vi "MasterStateController.vi"(1 "Selected State (In)":string) -> (0 "Selected State (Out)":string)   [LabVIEW 2019]
uses:
  6eb6b6c3-9e30-4625-8a84-628f4f349f2d.vi
  6eb6b6c3-9e30-4625-8a84-628f4f349f2d.vi/f3f6f8f9-418a-4164-be9e-b0b809c44121.vi
  dsdata.vi
  constants.vi
  outputs.vi
  <vilib>/Rock Robotics/Network Tables/NT Write Value.vi
  <vilib>/Rock Robotics/Network Tables/NT Write String.vi
panel:
  out "State Index":i32
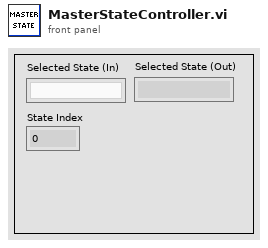
[diagram p1: front panel]
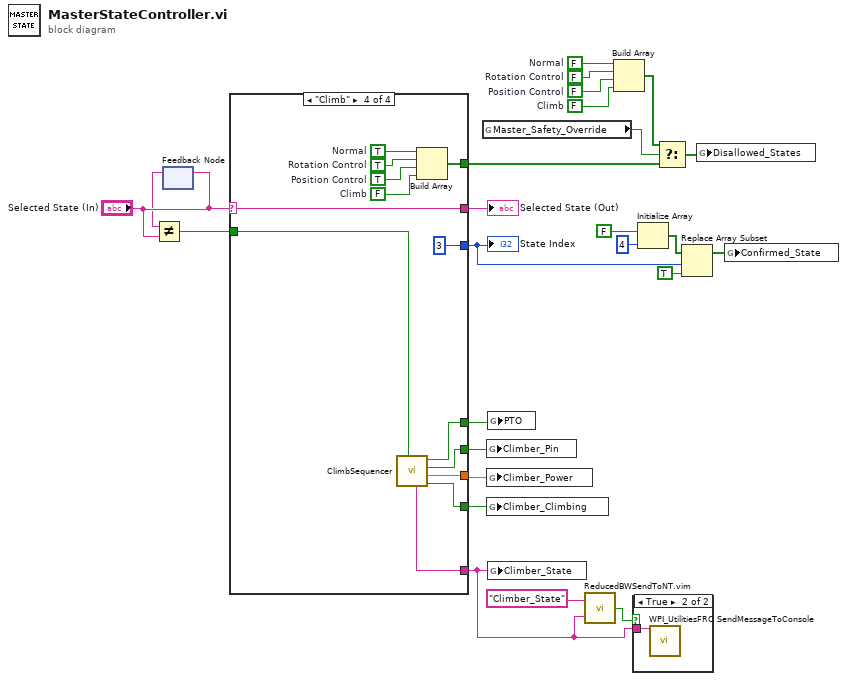
[diagram p0: block diagram]
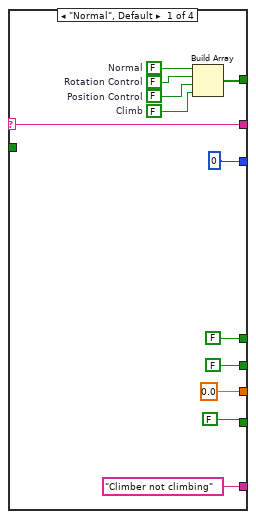
[diagram p3: hidden frame]
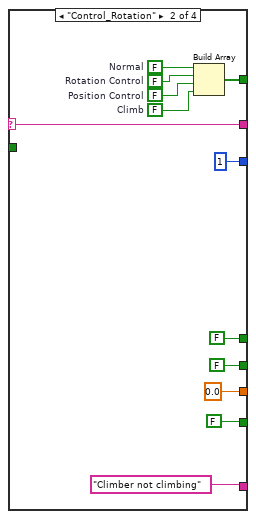
[diagram p4: hidden frame]
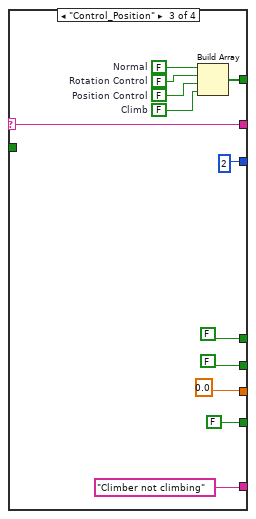
[diagram p5: hidden frame]
diagram:
  w12 = FALSE  # Climb
  w14 = FALSE  # Rotation Control
  w13 = FALSE  # Position Control
  w15 = FALSE  # Normal
  n1 = feedback-in #1("Selected State (In)") -> ()
  n2 = feedback #1() -> (w6:string)  [unwired: 1 in]
  n3 = Not Equal?(x=w6, y="Selected State (In)") -> (x != y?=w5:bool)
  n4 = case shown="\"Climb\"" "Selected State (In)" {
    selector: "Selected State (In)" -> [w36 w48 w61 w73]
    tunnel: [0 ("Index") 1 ("Index") 2 ("Index") 3 ("Index")] -> w22
    tunnel: [w36 w48 w61 w73] -> w19
    tunnel: [0.0 ("Climber_Power") 0.0 ("Climber_Power") 0.0 ("Climber_Power") w64] -> w4
    tunnel: [FALSE FALSE FALSE w63] -> w18
    tunnel: [FALSE FALSE FALSE w62] -> w17
    tunnel: ["Climber not climbing" "Climber not climbing" "Climber not climbing" w66] -> w1
    tunnel: [FALSE FALSE FALSE ("Flapper_Flapping") w65] -> w16
    tunnel: [w26 w38 w50 w68] -> w9
    tunnel: w5 -> [_ _ _ w67]
    frame "Normal", Default {
      w27 = FALSE  # Climb
      w29 = FALSE  # Rotation Control
      w28 = FALSE  # Position Control
      w30 = FALSE  # Normal
      n5 = Build Array(w30, w29, w28, w27) -> (w26:bool[])
    }
    frame "Control_Rotation" {
      w39 = FALSE  # Climb
      w41 = FALSE  # Rotation Control
      w40 = FALSE  # Position Control
      w42 = FALSE  # Normal
      n6 = Build Array(w42, w41, w40, w39) -> (w38:bool[])
    }
    frame "Control_Position" {
      w51 = FALSE  # Climb
      w53 = FALSE  # Rotation Control
      w52 = FALSE  # Position Control
      w54 = FALSE  # Normal
      n7 = Build Array(w54, w53, w52, w51) -> (w50:bool[])
    }
    frame "Climb" {
      w69 = FALSE  # Climb
      w71 = TRUE  # Rotation Control
      w70 = TRUE  # Position Control
      w72 = TRUE  # Normal
      n8 = call "ClimbSequencer.vi"("Reinit"=w67) -> ("Climber Climbing"=w65:bool, "Climber Power"=w64:dbl, "Climber Pin"=w63:bool, "PTO"=w62:bool, "Climber Step"=w66:string)  [unwired: 6 in]
      n9 = Build Array(w72, w71, w70, w69) -> (w68:bool[])
    }
  }
  "State Index" <- w22
  "Selected State (Out)" <- w19
  n10 = global read "dsdata.vi" "Master_Safety_Override"() -> (w11:bool)
  n11 = global write "outputs.vi" "Climber_Pin"(w18) -> ()
  n12 = global write "outputs.vi" "Climber_Power"(w4) -> ()
  n13 = global write "outputs.vi" "Climber_Climbing"(w16) -> ()
  n14 = global write "outputs.vi" "PTO"(w17) -> ()
  n15 = global write "outputs.vi" "Climber_State"(w1) -> ()
  n16 = call "ReducedBWSendToNT.vim"("Value In"=w1, "NT Name"="Climber_State" ("Name")) -> ("Value Changed"=w3:bool)
  n17 = Build Array(w15, w14, w13, w12) -> (w10:bool[])
  n18 = case shown="True" w3 {
    tunnel: w1 -> [_ w75]
    frame False {
    }
    frame True {
      n19 = call <vilib>:"WPI_UtilitiesFRC SendMessageToConsole.vi"("Message"=w75) -> ()  [unwired: 14 in, 1 out]
    }
  }
  n20 = Initialize Array(FALSE, 4 ("dimension size")) -> (w23:bool[])
  n21 = Select(t=w10, s=w11, f=w9) -> (s? t:f=w8:bool[])
  n22 = Replace Array Subset(array=w23, new element=TRUE ("new element/subarray"), index=w22) -> (w20:bool[])
  n23 = global write "constants.vi" "Disallowed_States"(w8) -> ()
  n24 = global write "outputs.vi" "Confirmed_State"(w20) -> ()
